vi "停止后释放.vi"(6 "Queue In":T1, 8 "error in (no error)":errorcluster) -> (0 "error out":errorcluster)   [LabVIEW 2015]
uses:
  Global/SeverGlobal.vi
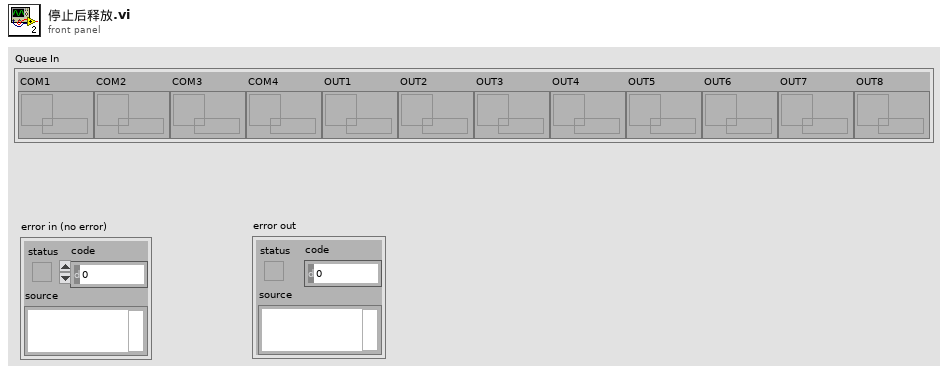
[diagram p1: front panel]
types:
  T1 = typedef "队列.ctl" = cluster{"COM1":refnum<queue>, "COM2":refnum<queue>, "COM3":refnum<queue>, "COM4":refnum<queue>, "OUT1":refnum<queue>, "OUT2":refnum<queue>, "OUT3":refnum<queue>, "OUT4":refnum<queue>, "OUT5":refnum<queue>, "OUT6":refnum<queue>, "OUT7":refnum<queue>, "OUT8":refnum<queue>}
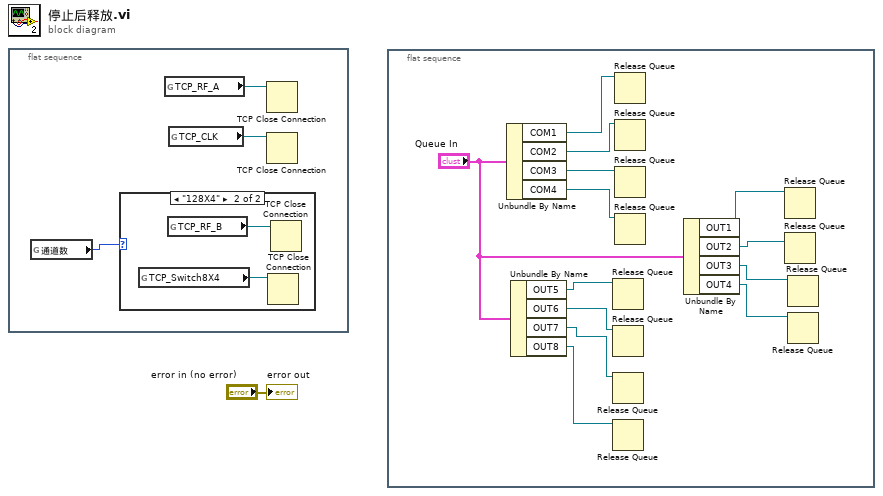
[diagram p0: block diagram]
diagram:
  n1 = flat-sequence {
    frame #0 {
      n2 = global read "SeverGlobal.vi" "通道数"() -> (w2:enum16{"64X4", "128X4"})
      n3 = case shown="\"128X4\"" w2 {
        frame "64X4", Default {
        }
        frame "128X4" {
          n4 = global read "SeverGlobal.vi" "TCP_Switch8X4"() -> (w5:refnum<k5>)
          n5 = global read "SeverGlobal.vi" "TCP_RF_B"() -> (w6:refnum<k5>)
          n6 = TCP Close Connection(connection ID=w5) -> ()  [unwired: 2 in, 2 out]
          n7 = TCP Close Connection(connection ID=w6) -> ()  [unwired: 2 in, 2 out]
        }
      }
      n8 = global read "SeverGlobal.vi" "TCP_RF_A"() -> (w4:refnum<k5>)
      n9 = global read "SeverGlobal.vi" "TCP_CLK"() -> (w3:refnum<k5>)
      n10 = TCP Close Connection(connection ID=w4) -> ()  [unwired: 2 in, 2 out]
      n11 = TCP Close Connection(connection ID=w3) -> ()  [unwired: 2 in, 2 out]
    }
  }
  n12 = flat-sequence {
    frame #0 {
      n13 = Unbundle By Name("Queue In") -> ("COM1"=w19:refnum<queue>, "COM2"=w18:refnum<queue>, "COM3"=w17:refnum<queue>, "COM4"=w16:refnum<queue>)
      n14 = Unbundle By Name("Queue In") -> ("OUT5"=w15:refnum<queue>, "OUT6"=w14:refnum<queue>, "OUT7"=w13:refnum<queue>, "OUT8"=w12:refnum<queue>)
      n15 = Release Queue(queue=w15) -> ()  [unwired: 2 in, 3 out]
      n16 = Release Queue(queue=w14) -> ()  [unwired: 2 in, 3 out]
      n17 = Release Queue(queue=w13) -> ()  [unwired: 2 in, 3 out]
      n18 = Release Queue(queue=w12) -> ()  [unwired: 2 in, 3 out]
      n19 = Release Queue(queue=w19) -> ()  [unwired: 2 in, 3 out]
      n20 = Release Queue(queue=w18) -> ()  [unwired: 2 in, 3 out]
      n21 = Release Queue(queue=w17) -> ()  [unwired: 2 in, 3 out]
      n22 = Release Queue(queue=w16) -> ()  [unwired: 2 in, 3 out]
      n23 = Unbundle By Name("Queue In") -> ("OUT1"=w10:refnum<queue>, "OUT2"=w9:refnum<queue>, "OUT3"=w8:refnum<queue>, "OUT4"=w7:refnum<queue>)
      n24 = Release Queue(queue=w10) -> ()  [unwired: 2 in, 3 out]
      n25 = Release Queue(queue=w9) -> ()  [unwired: 2 in, 3 out]
      n26 = Release Queue(queue=w8) -> ()  [unwired: 2 in, 3 out]
      n27 = Release Queue(queue=w7) -> ()  [unwired: 2 in, 3 out]
    }
  }
  "error out" <- "error in (no error)"
